vi "Parse Remote Terminal.vi"(8 "error in (no error)":errorcluster, 11 "Single RT XML Node":refnum<k20>) -> (0 "error out":errorcluster, 3 "Single RT":refnum<class "Remote Terminal.lvclass">[](array[class]))   [LabVIEW 2016]
doc: "Retrieves all the Remote Terminals defined for a single bus in XML."
uses:
  Remote Terminal/Remote Terminal.lvclass
  <vilib>/xml/NI_XML.lvlib
  Remote Terminal/TypeDefs/RT Configuration.ctl
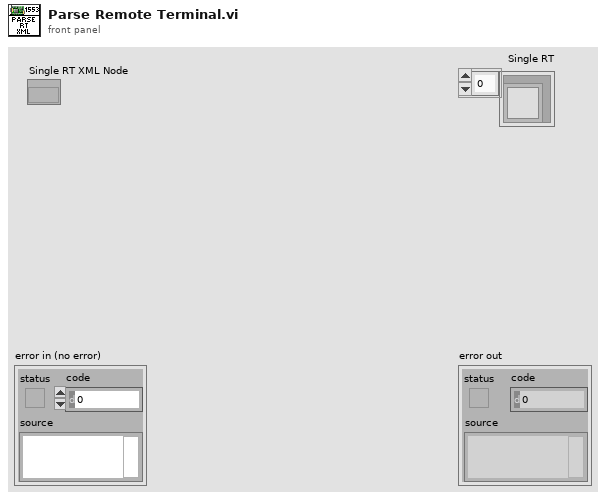
[diagram p1: front panel]
types:
  T1 = typedef "BCI-1553 API.lvlib/Remote Terminal.lvclass/RT Configuration.ctl" = cluster{"RT-RT TimeOut (us)":u8, "Inhibit Bus A":bool, "Inhibit Bus B":bool, "Broadcast CMD Invalid":bool, "UnDef MCs Invalid":bool, "Notice 2 Data Storage":bool, "SMCP":bool, "Temp RX Buffer":bool, "Alt BIT Enable":bool, "Auto Bus Shutdown":bool, "MC 17 Sync":u8, "MC 16 SR Reset":bool, "MC 8 Reset":bool}
  T2 = typedef "BCI-1553 API.lvlib/Remote Terminal.lvclass/Command Configuration.ctl" = cluster{"Command Type":T3, "Mode Code ID (1-32)":u16, "SubAddress (1-30)":u16, "Word Count (1-32)":u16, "Illegal Command":bool, "Broadcast":bool, "Data":u16[], "Data Fields":T4[]}
  T3 = typedef "BCI-1553 API.lvlib/Remote Terminal.lvclass/Command Type.ctl" = enum16{"Transmit", "Receive", "Mode Code Tx", "Mode Code Rx"}
  T4 = typedef "BCI-1553 API.lvlib/1553 SubComponent.lvclass/Parameter Table Data.ctl" = cluster{"Parameter Name":string, "Base Word":u16, "Address":u16, "Value":u64, "Mask":u16[], "Scaling Info":T5}
  T5 = typedef "BCI-1553 API.lvlib/1553 SubComponent.lvclass/Scaling Information.ctl" = cluster{"Bit Offset":i32, "Bit Count":i32, "LSB Resolution":dbl, "2's Complement":bool, "Big Endian":bool, "Sign Bit":bool}
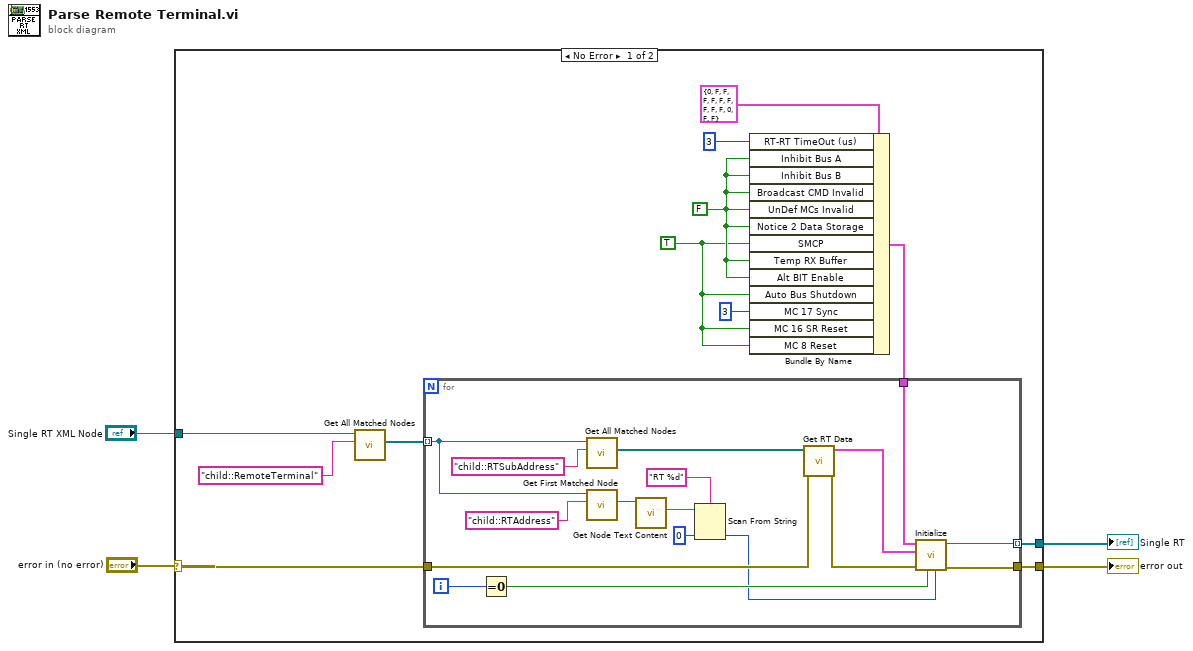
[diagram p0: block diagram]
diagram:
  n1 = case shown="No Error" "error in (no error)" {
    selector: "error in (no error)" -> [w6 w34]
    tunnel: [w16 w34] -> w3
    tunnel: "Single RT XML Node" -> [w14 _]
    tunnel: [w15 _] -> w1
    frame No Error {
      w7 = TRUE ("SMCP")
      w9 = FALSE ("UnDef MCs Invalid")
      n2 = call <vilib>:"Get All Matched Nodes.vi"("XPath expression"="child::RemoteTerminal", "node in"=w14) -> ("node result array"=w5:refnum<k20>[])  [unwired: 7 in, 2 out]
      n3 = Bundle By Name(cluster=T1 {"RT-RT TimeOut (us)"=0, "Inhibit Bus A"=FALSE, "Inhibit Bus B"=FALSE, "Broadcast CMD Invalid"=FALSE, "UnDef MCs Invalid"=FALSE, "Notice 2 Data Storage"=FALSE, "SMCP"=FALSE, "Temp RX Buffer"=FALSE, "Alt BIT Enable"=FALSE, "Auto Bus Shutdown"=FALSE, "MC 17 Sync"=0, "MC 16 SR Reset"=FALSE, "MC 8 Reset"=FALSE} ("RT Configuration"), "RT-RT TimeOut (us)"=u8 3, "Inhibit Bus A"=w9, "Inhibit Bus B"=w9, "Broadcast CMD Invalid"=w9, "UnDef MCs Invalid"=w9, "Notice 2 Data Storage"=w9, "SMCP"=w7, "Temp RX Buffer"=w9, "Alt BIT Enable"=w9, "Auto Bus Shutdown"=w7, "MC 17 Sync"=u8 3, "MC 16 SR Reset"=w7, "MC 8 Reset"=w7) -> (w11:T1)
      n4 = for {
        tunnel: [w26] -> w15 mode=indexing
        tunnel: w11 -> [w32]
        tunnel: w6 -> [w28]
        tunnel: [w33] -> w16
        tunnel: w5 -> [w24] mode=indexing
        i -> [w22]
        n5 = Equal To 0?(x=w22) -> (x = 0?=w21:bool)
        n6 = call <vilib>:"Get All Matched Nodes.vi"("XPath expression"="child::RTSubAddress", "node in"=w24) -> ("node result array"=w30:refnum<k20>[])  [unwired: 7 in, 2 out]
        n7 = call <vilib>:"Get First Matched Node.vi"("XPath expression"="child::RTAddress", "node in"=w24) -> ("node result"=w23:refnum<k20>)  [unwired: 7 in, 2 out]
        n8 = call <vilib>:"Get Node Text Content.vi"("node in"=w23) -> ("node text"=w20:string)  [unwired: 8 in, 2 out]
        n9 = Scan From String(format string="RT %d", input string=w20, default 1=u8 0 ("default value 1")) -> (output 1=w18:u8)  [unwired: 2 in, 3 out]
        n10 = call "Get RT Data.vi"("error in (no error)"=w28, "RT SubAddresses XML Ref"=w30) -> ("error out"=w27:errorcluster, "SubAddress Configurations"=w29:T2[])  [unwired: 8 in]
        n11 = call "Initialize.vi"("RT Address (0-30)"=w18, "RT 1?"=w21, "error in (no error)"=w27, "Commands"=w29, "RT Configuration"=w32) -> ("error out"=w33:errorcluster, "Remote Terminal out"=w26:refnum<class "Remote Terminal.lvclass">)  [unwired: 5 in]
      }
    }
    frame Error {
    }
  }
  "error out" <- w3
  "Single RT" <- w1
